vi "NameData_Array Data.vi"(8 "Error":errorcluster, 11 "Array Variant":variant) -> (0 "Error Out":errorcluster, 2 "ArrayElement Out":variant, 3 "Dim Sizes Out":u32[](array[numeric]), 5 "Data String Out":string)   [LabVIEW 2015]
uses:
  <vilib>/Utility/VariantDataType/VariantType.lvlib
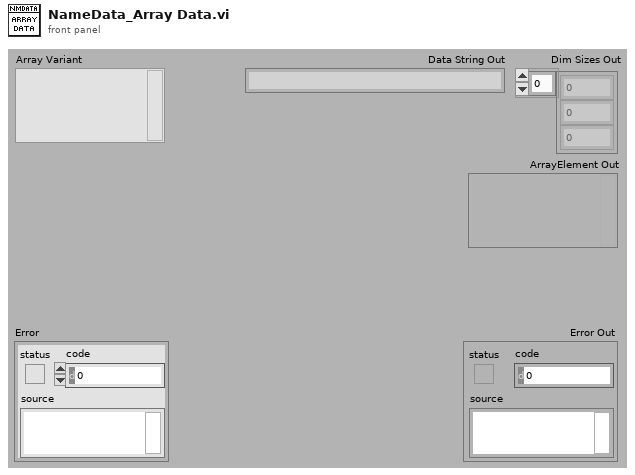
[diagram p1: front panel]
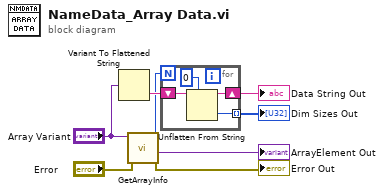
[diagram p0: block diagram]
diagram:
  n1 = Variant To Flattened String(Variant="Array Variant") -> (data string=w4:string)  [unwired: 1 out]
  n2 = call <vilib>:"GetArrayInfo.vi"("error in (no error)"="Error", "Variant"="Array Variant") -> ("error out"=→"Error Out":errorcluster, "ArrayElement"=→"ArrayElement Out":variant, "NDims"=w3:i32)  [unwired: 6 in, 1 out]
  n3 = for {
    N: w3 -> [_]
    shift-right: [w10] -> w5
    shift-left: w4 -> [w11]
    tunnel: [w9] -> w6 mode=indexing
    n4 = Unflatten From String(type=u32 0, binary string=w11) -> (rest of the binary string=w10:string, value=w9:u32)  [unwired: 3 in, 1 out]
  }
  "Dim Sizes Out" <- w6
  "Data String Out" <- w5
